vi "Status_asyncvarsMgr.vi"(7 "action":T3(ring), 8 "error in (no error)":errorcluster, 9 "value":string, 10 "var":string, 11 "Database RefNum in":T1) -> (0 "enabled":bool, 1 "found":bool, 2 "vars":T2[](array[typedef]), 3 "names":string[](array[string]))   [LabVIEW 2016]
uses:
  Status_VarsStruct.ctl
  DBSHAND/private/vis/DatabaseHand_RefNum.ctl
panel:
  out "all":bool
  in  "var":T2
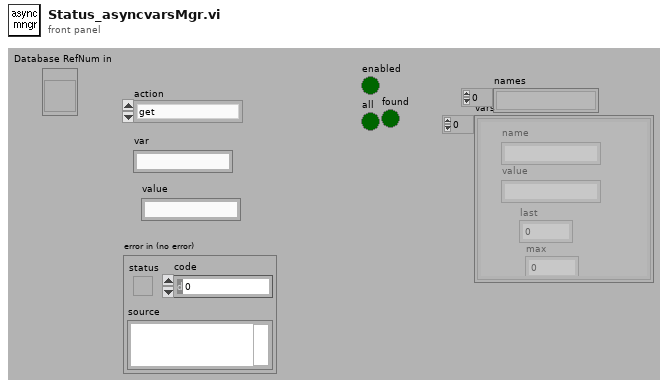
[diagram p1: front panel]
types:
  T1 = typedef "DatabaseHand_RefNum.ctl" = refnum<vi>
  T2 = typedef "Status_VarsStruct.ctl" = cluster{"name":string, "value":string, "last":u32, "max":u32}
  T3 = enum16{"get", "send", "delete", "add", "clean", "send_all", "send_on", "send_off"}
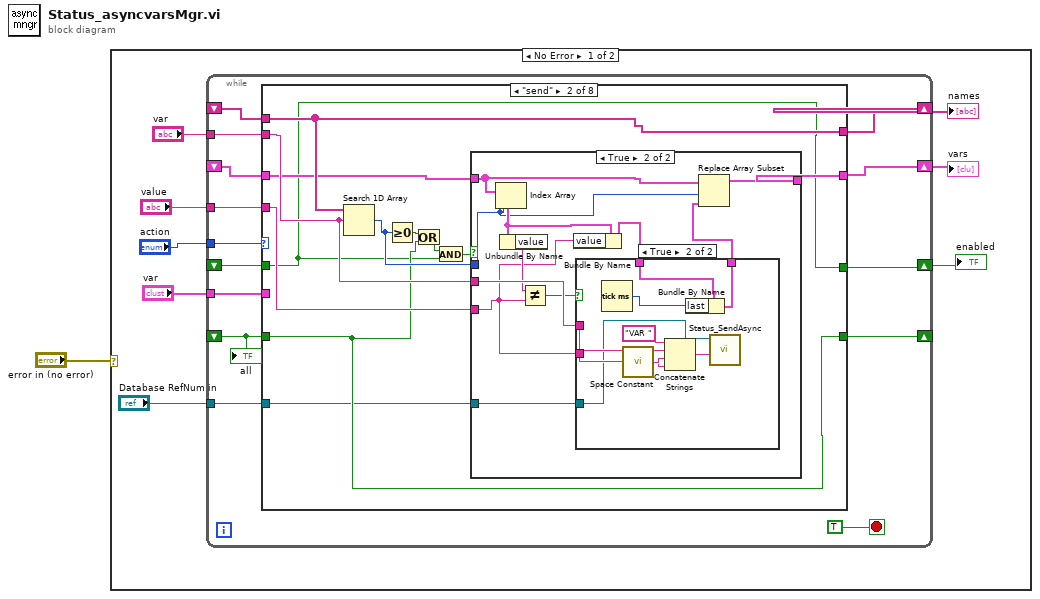
[diagram p0: block diagram]
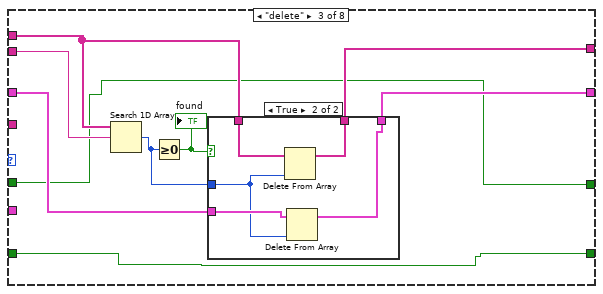
[diagram p5: hidden frame]
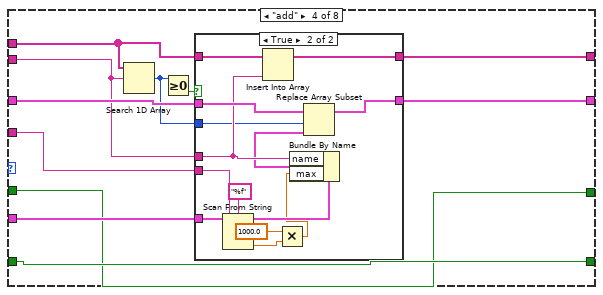
[diagram p7: hidden frame]
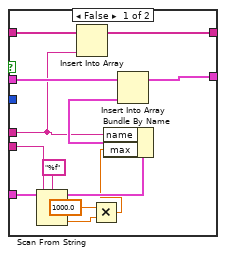
[diagram p8: hidden frame]
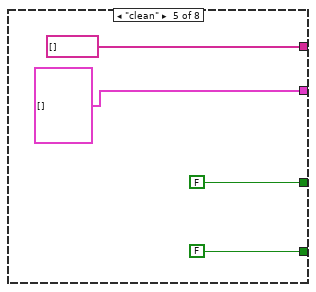
[diagram p9: hidden frame]
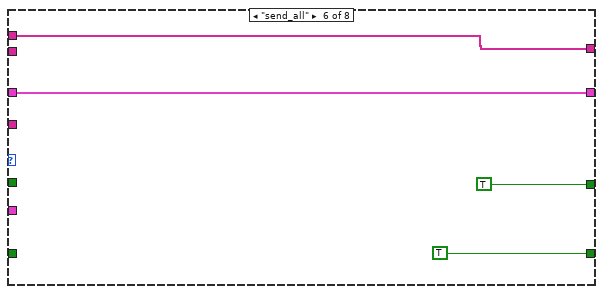
[diagram p10: hidden frame]
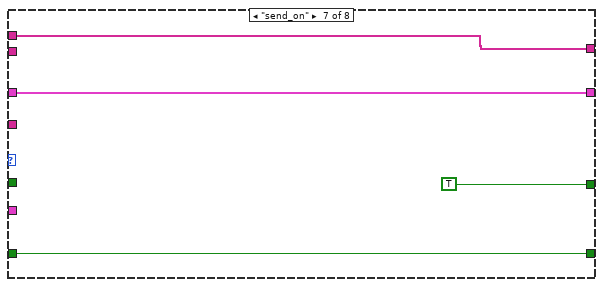
[diagram p11: hidden frame]
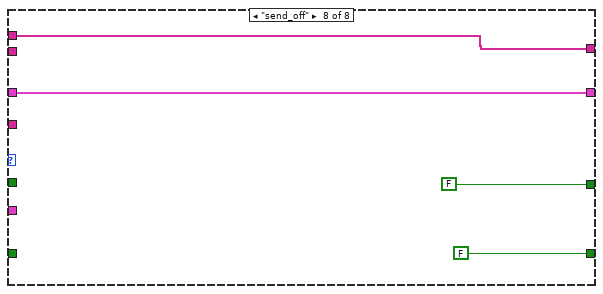
[diagram p12: hidden frame]
diagram:
  n1 = case shown="No Error" "error in (no error)" {
    frame No Error {
      n2 = while {
        tunnel: "action" -> [w22]
        shift-right: [w18] -> w4
        shift-left: _ -> [w17]
        tunnel: "var" -> [w21]
        tunnel: "var" -> [w20]
        tunnel: "value" -> [w19]
        shift-right: [w16] -> w5
        shift-left: _ -> [w15]
        shift-right: [w14] -> _
        shift-left: _ -> [w13]
        shift-right: [w12] -> w2
        shift-left: _ -> [w11]
        tunnel: "Database RefNum in" -> [w10]
        stop <- TRUE stop-if-true
        n3 = case shown="\"send\"" w22 {
          tunnel: w21 -> [_ _ _ w88 _ _ _ _]
          tunnel: w20 -> [_ w37 w64 w81 _ _ _ _]
          tunnel: w19 -> [_ w36 _ w87 _ _ _ _]
          tunnel: [w26 w33 w65 w86 T2[] [] ("vars") w120 w124 w128] -> w18
          tunnel: w17 -> [w26 w34 w68 w85 _ w120 w124 w128]
          tunnel: [w27 w39 w66 w84 string[] [] w121 w125 w129] -> w16
          tunnel: w15 -> [w27 w39 w69 w83 _ w121 w125 w129]
          tunnel: [w25 w32 w63 w80 FALSE TRUE w123 FALSE] -> w14
          tunnel: w13 -> [w25 w32 w63 w80 _ _ w123 _]
          tunnel: [w24 w29 w62 w79 FALSE TRUE TRUE FALSE] -> w12
          tunnel: w11 -> [w24 w29 w62 w79 _ _ _ _]
          tunnel: w10 -> [_ w28 _ _ _ _ _ _]
          frame "get", Default {
          }
          frame "send" {
            n4 = Search 1D Array(1D array=w39, element=w37) -> (index of element=w35:i32)  [unwired: 1 out]
            n5 = Greater Or Equal To 0?(x=w35) -> (x >= 0?=w38:bool)
            n6 = Or(x=w38, y=w32) -> (x .or. y?=w30:bool)
            n7 = And(x=w30, y=w29) -> (x .and. y?=w31:bool)
            n8 = case shown="True" w31 {
              tunnel: w37 -> [_ w47]
              tunnel: w36 -> [_ w45]
              tunnel: w35 -> [_ w49]
              tunnel: w34 -> [w40 w50]
              tunnel: [w40 w48] -> w33
              tunnel: w28 -> [_ w42]
              frame False {
              }
              frame True {
                n9 = Index Array(array=w50, index=w49) -> (element=w51:T2)
                n10 = Unbundle By Name(w51) -> ("value"=w46:string)
                n11 = Not Equal?(x=w46, y=w45) -> (x != y?=w44:bool)
                n12 = Bundle By Name(cluster=w51, "value"=w45) -> (w43:T2)
                n13 = case shown="True" w44 {
                  tunnel: w47 -> [_ w60]
                  tunnel: w45 -> [_ w58]
                  tunnel: w43 -> [w52 w56]
                  tunnel: w42 -> [_ w55]
                  tunnel: [w52 w54] -> w41
                  frame False {
                  }
                  frame True {
                    n14 = Tick Count (ms)() -> (millisecond timer value=w53:u32)
                    n15 = call <vilib>:"Space Constant.vi"() -> ("String"=w59:string)
                    n16 = Concatenate Strings("VAR " ("string"), w60, w59, w58) -> (w57:string)
                    n17 = Bundle By Name(cluster=w56, "last"=w53) -> (w54:T2)
                    n18 = call "Status_SendAsync.vi"("Message"=w57, "Database RefNum in"=w55) -> ()  [unwired: 1 in, 9 out]
                  }
                }
                n19 = Replace Array Subset(array=w50, new element=w41, index=w49) -> (w48:T2[])
              }
            }
          }
          frame "delete" {
            n20 = Search 1D Array(1D array=w69, element=w64) -> (index of element=w67:i32)  [unwired: 1 out]
            n21 = Greater Or Equal To 0?(x=w67) -> (x >= 0?=w70:bool)
            "found" <- w70
            n22 = case shown="True" w70 {
              tunnel: w69 -> [w72 w77]
              tunnel: w68 -> [w71 w75]
              tunnel: w67 -> [_ w73]
              tunnel: [w72 w76] -> w66
              tunnel: [w71 w74] -> w65
              frame False {
              }
              frame True {
                n23 = Delete From Array(array=w77, index=w73) -> (array with subset deleted=w76:string[])  [unwired: 1 in, 1 out]
                n24 = Delete From Array(array=w75, index=w73) -> (array with subset deleted=w74:T2[])  [unwired: 1 in, 1 out]
              }
            }
          }
          frame "add" {
            n25 = Search 1D Array(1D array=w83, element=w81) -> (index of element=w78:i32)  [unwired: 1 out]
            n26 = Greater Or Equal To 0?(x=w78) -> (x >= 0?=w82:bool)
            n27 = case shown="True" w82 {
              tunnel: w88 -> [w100 w113]
              tunnel: w87 -> [w93 w107]
              tunnel: [w98 w112] -> w86
              tunnel: w85 -> [w97 w111]
              tunnel: w81 -> [w94 w108]
              tunnel: [w96 w110] -> w84
              tunnel: w83 -> [w95 w109]
              tunnel: w78 -> [_ w101]
              frame False {
                n28 = Scan From String(format string="%f", input string=w93) -> (output 1=w91:dbl)  [unwired: 2 in, 4 out]
                n29 = Insert Into Array(array=w95, new element=w94) -> (w96:string[])  [unwired: 1 in]
                n30 = Multiply(x=1000.0, y=w91) -> (x*y=w89:dbl)
                n31 = Bundle By Name(cluster=w100, "name"=w94, "max"=w89) -> (w99:T2)
                n32 = Insert Into Array(array=w97, new element=w99) -> (w98:T2[])  [unwired: 1 in]
              }
              frame True {
                n33 = Scan From String(format string="%f", input string=w107) -> (output 1=w105:dbl)  [unwired: 2 in, 4 out]
                n34 = Insert Into Array(array=w109, new element=w108) -> (w110:string[])  [unwired: 1 in]
                n35 = Multiply(x=1000.0, y=w105) -> (x*y=w103:dbl)
                n36 = Bundle By Name(cluster=w113, "name"=w108, "max"=w103) -> (w102:T2)
                n37 = Replace Array Subset(array=w111, new element=w102, index=w101) -> (w112:T2[])
              }
            }
          }
          frame "clean" {
          }
          frame "send_all" {
          }
          frame "send_on" {
          }
          frame "send_off" {
          }
        }
        "all" <- w13
      }
      "enabled" <- w2
      "vars" <- w4
      "names" <- w5
    }
    frame Error {
    }
  }
